vi "HW_6p1_Task1_gamagetd.vi"() -> ()   [LabVIEW 2016]
panel:
  out "Final concentraiton of A":dbl
  out "Final concentration of B":dbl
  out "Time for desired C":dbl
  out "C final concentration (mo/L)":dbl
  in  "C target concentration (mol/L)":dbl
  in  "k3= 9.6E-13 (L4/(mol4*min))":dbl
  in  "k2= 3.44E-7 (L/(mol*min))":dbl
  in  "k1= 4.6E-5 (L2/(mol2*min))":dbl
  in  "B initial concentration(CBi)":dbl
  in  "A initial concentration(CAi)":dbl
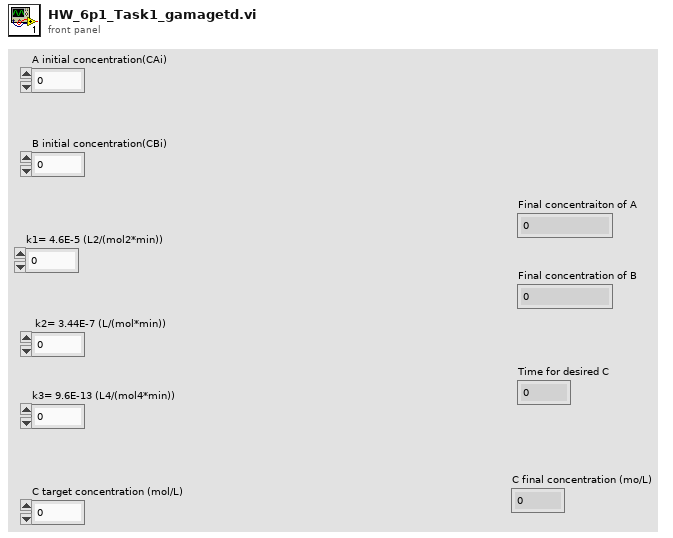
[diagram p1: front panel]
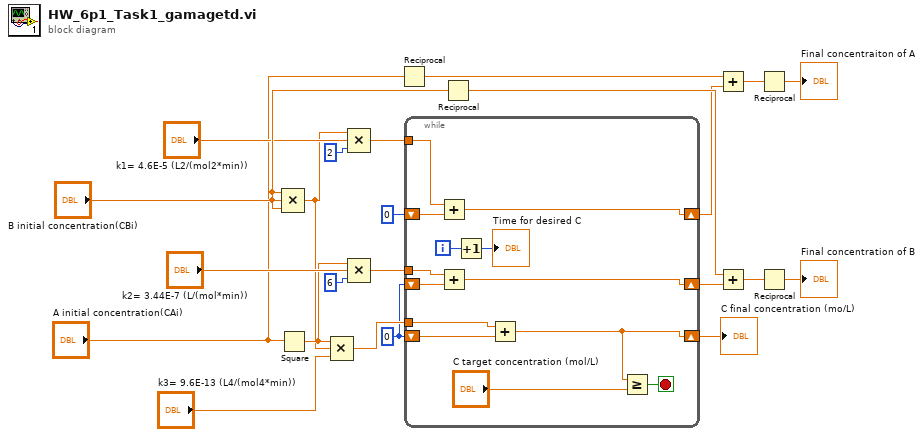
[diagram p0: block diagram]
diagram:
  w17 = 0
  n1 = Square(x="A initial concentration(CAi)") -> (x^2=w18:dbl)
  n2 = Compound Arithmetic op=MULTIPLY("B initial concentration(CBi)", "B initial concentration(CBi)", "B initial concentration(CBi)") -> (w8:dbl)
  n3 = Compound Arithmetic op=MULTIPLY(w18, w8, "k3= 9.6E-13 (L4/(mol4*min))") -> (w22:dbl)
  n4 = Compound Arithmetic op=MULTIPLY(w8, "k1= 4.6E-5 (L2/(mol2*min))", 2) -> (w6:dbl)
  n5 = Compound Arithmetic op=MULTIPLY(w18, "k2= 3.44E-7 (L/(mol*min))", 6) -> (w16:dbl)
  n6 = Reciprocal(x="A initial concentration(CAi)") -> (1/x=w4:dbl)
  n7 = while {
    shift-right: [w34] -> w21
    shift-left: w17 -> [w36]
    tunnel: w22 -> [w35]
    shift-right: [w27] -> w13
    shift-left: w17 -> [w29]
    tunnel: w16 -> [w28]
    shift-right: [w24] -> w3
    shift-left: 0 -> [w25]
    tunnel: w6 -> [w26]
    i -> [w31]
    stop <- w32 stop-if-true
    n8 = Add(x=w26, y=w25) -> (x+y=w24:dbl)
    n9 = Add(x=w28, y=w29) -> (x+y=w27:dbl)
    n10 = Increment(x=w31) -> (x+1=→"Time for desired C":i32)
    n11 = Add(x=w35, y=w36) -> (x+y=w34:dbl)
    n12 = Greater Or Equal?(x=w34, y="C target concentration (mol/L)") -> (x >= y?=w32:bool)
  }
  "C final concentration (mo/L)" <- w21
  n13 = Reciprocal(x="B initial concentration(CBi)") -> (1/x=w14:dbl)
  n14 = Add(x=w4, y=w3) -> (x+y=w2:dbl)
  n15 = Add(x=w14, y=w13) -> (x+y=w12:dbl)
  n16 = Reciprocal(x=w2) -> (1/x=→"Final concentraiton of A":dbl)
  n17 = Reciprocal(x=w12) -> (1/x=→"Final concentration of B":dbl)
